vi "T_FlipFlop.vi"(10 "stop":bool, 11 "Toggle":bool) -> (2 "!Q":bool, 3 "Q":bool)   [LabVIEW 2012]
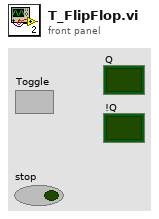
[diagram p1: front panel]
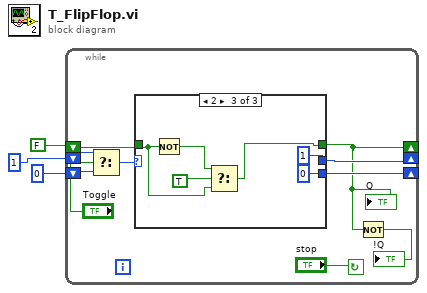
[diagram p0: block diagram]
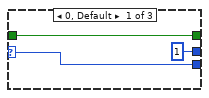
[diagram p2: hidden frame]
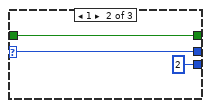
[diagram p3: hidden frame]
diagram:
  n1 = while {
    shift-right: [w10] -> _
    shift-left: 0 -> [w13]
    shift-right: [w7] -> _
    shift-left: FALSE ("Toggle") -> [w4]
    shift-right: [w9] -> _
    shift-left: 1 -> [w11]
    stop <- "stop" continue-if-true
    n2 = Select(t=w11, s="Toggle", f=w13) -> (s? t:f=w12:i32)
    n3 = case shown="2" w12 {
      selector: w12 -> [w15 w18 _]
      tunnel: [w16 w17 w20] -> w7
      tunnel: w4 -> [w16 w17 w21]
      tunnel: [w15 2 0] -> w10
      tunnel: [1 w18 1] -> w9
      frame 0, Default {
      }
      frame 1 {
      }
      frame 2 {
        n4 = Not(x=w21) -> (.not. x?=w22:bool)
        n5 = Select(t=w22, s=TRUE ("Toggle"), f=w21) -> (s? t:f=w20:bool)
      }
    }
    "Q" <- w7
    n6 = Not(x=w7) -> (.not. x?=→"!Q":bool)
  }
